vi "Init Error Loop.vi"(6 "Max File Size":i64=10485760, 8 "Error In":errorcluster, 9 "Application Errors":path, 10 "Error Log":path, 11 "Update Queue":refnum<queue>) -> (0 "Error Out":errorcluster)   [LabVIEW 2019, in "TSC Error.lvlib"]
doc: "Use this VI to set up the Error Loop Queue and initialize certain inputs.\n\nInputs:\n-Update Queue [queue ref] - this API will use a Queue with a cluster of string (message) and variant (data) to send a message to prompt the user if desired\n-Error Log [path] - the file path to the application's error log (if empty, will default to error.txt at the top level)\n-Application Errors [path] - the file path for custom errors for the application if applicable\n-Max File Size [I64] - define the maximum error log file size so that it doesn't grow indefinitely\n-error in\n\nOutputs:\n-error out\n\n<b>Code Developed By:</b>\nDaniel Coons\nTechnology Service Corporation\n1983 S Liberty Drive\nBloomington, IN 47403\nwww.tsc.com\\atcs"
uses:
  TSC Error.lvlib
  _Messages/ERROR_Init/ERROR_Init.lvclass
  C:/Development/Open Source/tsc-error-library/_Messages/Error/Error.lvclass
  _Messages/Error/Error.lvclass/Error.ctl
  _Messages/Error/Error.lvclass
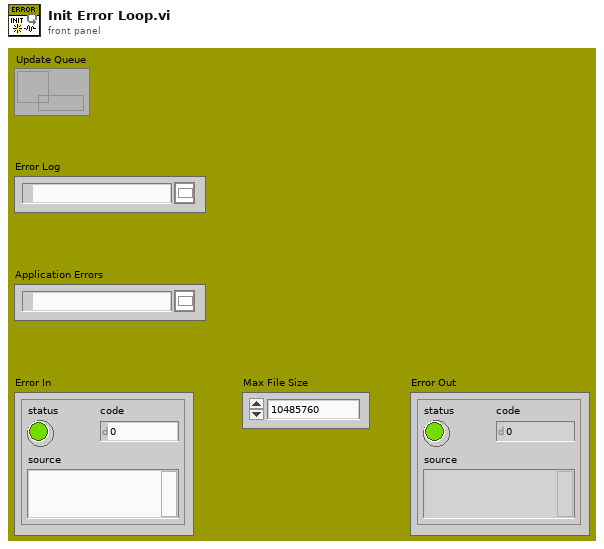
[diagram p1: front panel]
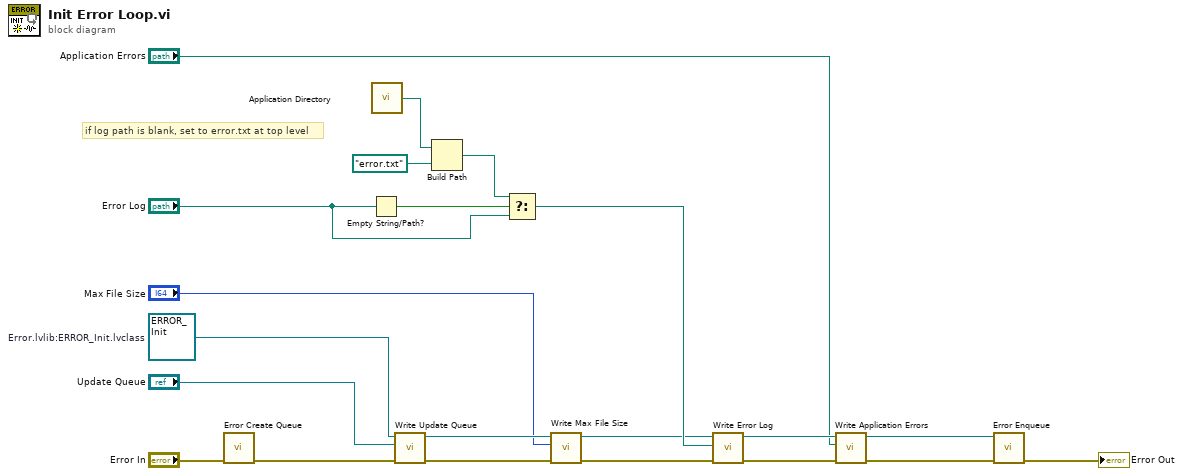
[diagram p0: block diagram]
diagram:
  w21 = refnum<class "ERROR_Init.lvclass"> refnum  # Error.lvlib:ERROR_Init.lvclass
  # "if log path is blank, set to error.txt at top level"
  n1 = call "Error Create Queue.vi"("error in (no error)"="Error In") -> ("error out"=w11:errorcluster)  [unwired: 8 in, 2 out]
  n2 = Empty String/Path?(string/path="Error Log") -> (empty?=w10:bool)
  n3 = call <vilib>:"Application Directory.vi"() -> ("Application Directory"=w7:path)
  n4 = call "Write Update Queue.vi"("error in (no error)"=w11, "Update Queue"="Update Queue", "Error in"=w21) -> ("error out"=w19:errorcluster, "Error out"=w3:refnum<class "ERROR_Init.lvclass">)  [unwired: 7 in]
  n5 = Build Path(base path=w7, name or relative path=path "error.txt") -> (appended path=w5:path)
  n6 = Select(t=w5, s=w10, f="Error Log") -> (s? t:f=w8:path)
  n7 = call "Write Max File Size.vi"("error in (no error)"=w19, "Max File Size"="Max File Size", "Error in"=w3) -> ("error out"=w4:errorcluster, "Error out"=w2:refnum<class "ERROR_Init.lvclass">)  [unwired: 7 in]
  n8 = call "Write Error Log.vi"("error in (no error)"=w4, "Error Log"=w8, "Error in"=w2) -> ("error out"=w17:errorcluster, "Error out"=w14:refnum<class "ERROR_Init.lvclass">)  [unwired: 7 in]
  n9 = call "Write Application Errors.vi"("error in (no error)"=w17, "Application Errors"="Application Errors", "Error in"=w14) -> ("error out"=w16:errorcluster, "Error out"=w15:refnum<class "ERROR_Init.lvclass">)  [unwired: 7 in]
  n10 = call "Error Enqueue.vi"("error in"=w16, "Error Message in"=w15) -> ("error out"=→"Error Out":errorcluster)  [unwired: 8 in, 1 out]
